vi "SDG60ConfPulse.vi"() -> ()   [LabVIEW 2018]
doc: "Selects the waveform shape, frequency, amplitude, offset, and phase for standard waveforms (including Sine, Square, Ramp, Pulse, DC and Arb).\n\nNotes: \nTo configure other parameters for pulse waveforms please run the Configure Pulse VI. \nTo configure noise waveform please run the Configure Noise VI.\nTo configure other parameters for arbitrary waveforms please run the Create Arbitrary Waveform. \nTo configure PRBS waveform please run the Configure PRBS Waveform VI."
panel:
  in  "Rise Edge (s)":dbl=50.0 format="%#.6f"
  in  "Pulse Width (s)":dbl=50.0 format="%#.6f"
  in  "Freq/Period (T:Freq)":bool=TRUE
  in  "Channel (1:Channel 1)":i32(ring)=1 items=["Channel 1"=1, "Channel 2"=2]
  in  "Delay (s)":dbl min=-360.0 max=360.0 format="%#.15g"
  in  "Offset (0.00 V)":dbl format="%#_15g"
  in  "Amplitude (1.0 Vpp)":dbl=0.1 format="%#.6f"
  in  "Frequency/Period (1 Hz/s)":dbl=1000.0 format="%#.16g"
  out "VISA resource name out":refnum<visa-resource-name>
  out "error out":errorcluster
  in  "error in (no error)":errorcluster
  in  "VISA resource name":refnum<visa-resource-name>="USB0::0xF4EC::0x1101::SDG6XEBC5R0119::INSTR"
  # "Select pulse using SDG60ConfSTDWFM\nThen use this vi to change parameters"
  # "0.1mV resolution"
  # "Range: 1 uHz-200 MHz\nRange: 20 ns-1 Ms\nInternally max res 10 digits for freq, 6 digits for period"
  # "TODO: pulse width not working\n    change between rise/fall edge\n    duty cycle/pulse width\n    amplitude/high level\n    offset/lowlevel"
  # "0.1mV resolution"
  # "Range : 0%-100%\n6 digit precision"
  # "Range: 0s- Pulse Period"
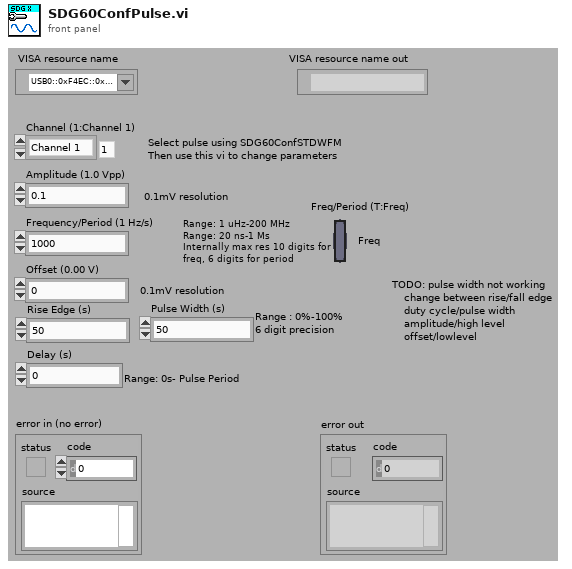
[diagram p1: front panel]
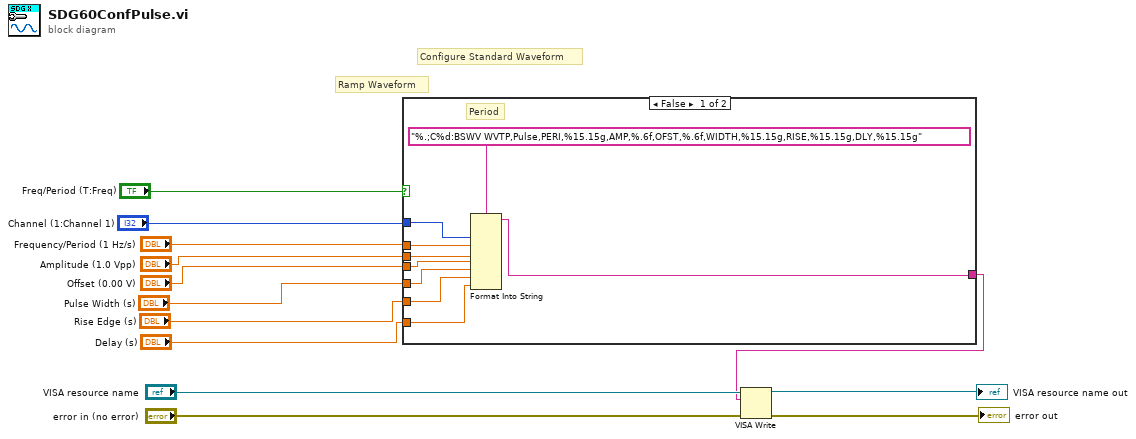
[diagram p0: block diagram]
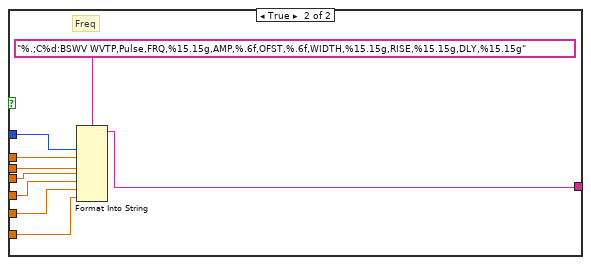
[diagram p2: hidden frame]
diagram:
  # "Ramp Waveform"
  # "Configure Standard Waveform"
  n1 = case shown="False" "Freq/Period (T:Freq)" {
    tunnel: [w21 w30] -> w11
    tunnel: "Channel (1:Channel 1)" -> [w20 w29]
    tunnel: "Frequency/Period (1 Hz/s)" -> [w19 w28]
    tunnel: "Amplitude (1.0 Vpp)" -> [w18 w27]
    tunnel: "Offset (0.00 V)" -> [w17 w26]
    tunnel: "Pulse Width (s)" -> [w16 w25]
    tunnel: "Rise Edge (s)" -> [w15 w24]
    tunnel: "Delay (s)" -> [w14 w23]
    frame False {
      # "Period"
      n2 = Format Into String(format string="%.;C%d:BSWV WVTP,Pulse,PERI,%15.15g,AMP,%.6f,OFST,%.6f,WIDTH,%15.15g,RISE,%15.15g,DLY,%15.15g", w20, w19, w18, w17, w16, w15, w14) -> (resulting string=w21:string)  [unwired: 2 in, 1 out]
    }
    frame True {
      # "Freq"
      n3 = Format Into String(format string="%.;C%d:BSWV WVTP,Pulse,FRQ,%15.15g,AMP,%.6f,OFST,%.6f,WIDTH,%15.15g,RISE,%15.15g,DLY,%15.15g", w29, w28, w27, w26, w25, w24, w23) -> (resulting string=w30:string)  [unwired: 2 in, 1 out]
    }
  }
  n4 = VISA Write(VISA resource name="VISA resource name", write buffer=w11, error in (no error)="error in (no error)") -> (VISA resource name out=→"VISA resource name out":refnum<visa-resource-name>, error out=→"error out":errorcluster)  [unwired: 1 out]
